vi "Climb_Motors.vi"(4 "Driver - Right Thumb":bool, 6 "Driver - Left Thumb":bool, 8 "Driver - Trigger":bool, 9 "Driver - Left Top left":bool, 10 "Driver - Right Top Right":bool) -> ()   [LabVIEW 2020]
uses:
  <vilib>/Rock Robotics/WPI/ThirdParty/Phoenix-LabVIEW/Motor Controller/Controls/CTRE_Phoenix_MotorControl_ControlMode.ctl
  <vilib>/Rock Robotics/Network Tables/NT Read String.vi
panel:
  in  "Traversal 2":dbl
  in  "Traversal 1":dbl
  in  "High 2":dbl
  in  "High 1":dbl
  in  "Mid 2":dbl=400000.0
  in  "Mid 1":dbl=400000.0
  in  "Low 2":dbl=150000.0
  in  "Low 1":dbl=150000.0
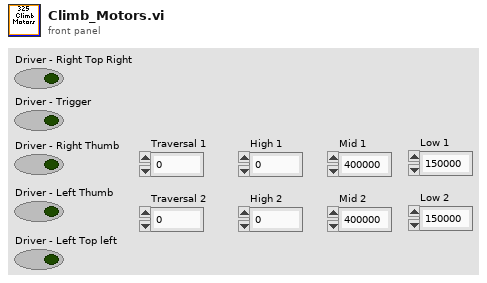
[diagram p1: front panel]
types:
  T1 = typedef "WPI_MotorControlDeviceRef.ctl" = cluster{"DeviceStatus":errorcluster, "Type":T2, "PWM":cluster{"PWM Channel":T3, "DeadBand":T4}, "CAN":cluster{"Device Number":u8, "SetOutput VI Ref":variant, "GetOutput VI Ref":variant, "Enable VI Ref":variant, "Disable VI Ref":variant, "Data":variant}, "Invert":bool, "DIO PWM":cluster{"PWM \"Enable\" Channel":T3, "DIOChannel":T5, "PWM Rate":dbl}}
  T2 = typedef "WPI_MotorControlType.ctl" = enum16{"PWM", "CAN", "DIO PWM"}
  T3 = typedef "FPGA_DIOPWMChannel.ctl" = enum8{"PWM 0", "PWM 1", "PWM 2", "PWM 3", "PWM 4", "PWM 5", "PWM 6", "PWM 7", "PWM 8", "PWM 9", "PWM MXP 0", "PWM MXP 1", "PWM MXP 2", "PWM MXP 3", "PWM MXP 4", "PWM MXP 5", "PWM MXP 6", "PWM MXP 7", "PWM MXP 8", "PWM MXP 9", "Invalid"}
  T4 = typedef "WPI_PWMDeadband.ctl" = cluster{"Name":string, "maxPositivePwm":i32, "minPositivePwm":i32, "centerPwm":i32, "maxNegativePwm":i32, "minNegativePwm":i32, "angularRange":u16}
  T5 = typedef "FPGA_DIOChannel.ctl" = enum8{"DIO 0", "DIO 1", "DIO 2", "DIO 3", "DIO 4", "DIO 5", "DIO 6", "DIO 7", "DIO 8", "DIO 9", "DIO MXP 0", "DIO MXP 1", "DIO MXP 2", "DIO MXP 3", "DIO MXP 4", "DIO MXP 5", "DIO MXP 6", "DIO MXP 7", "DIO MXP 8", "DIO MXP 9", "DIO MXP 10", "DIO MXP 11", "DIO MXP 12", "DIO MXP 13", "DIO MXP 14", "DIO MXP 15", "SPI Port CS1", "SPI Port CS2", "SPI Port CS3", "SPI Port MISO", "SPI Port MOSI", "Invalid"}
  T6 = typedef "CTRE_Phoenix_MotorControl_ControlMode.ctl" = u16
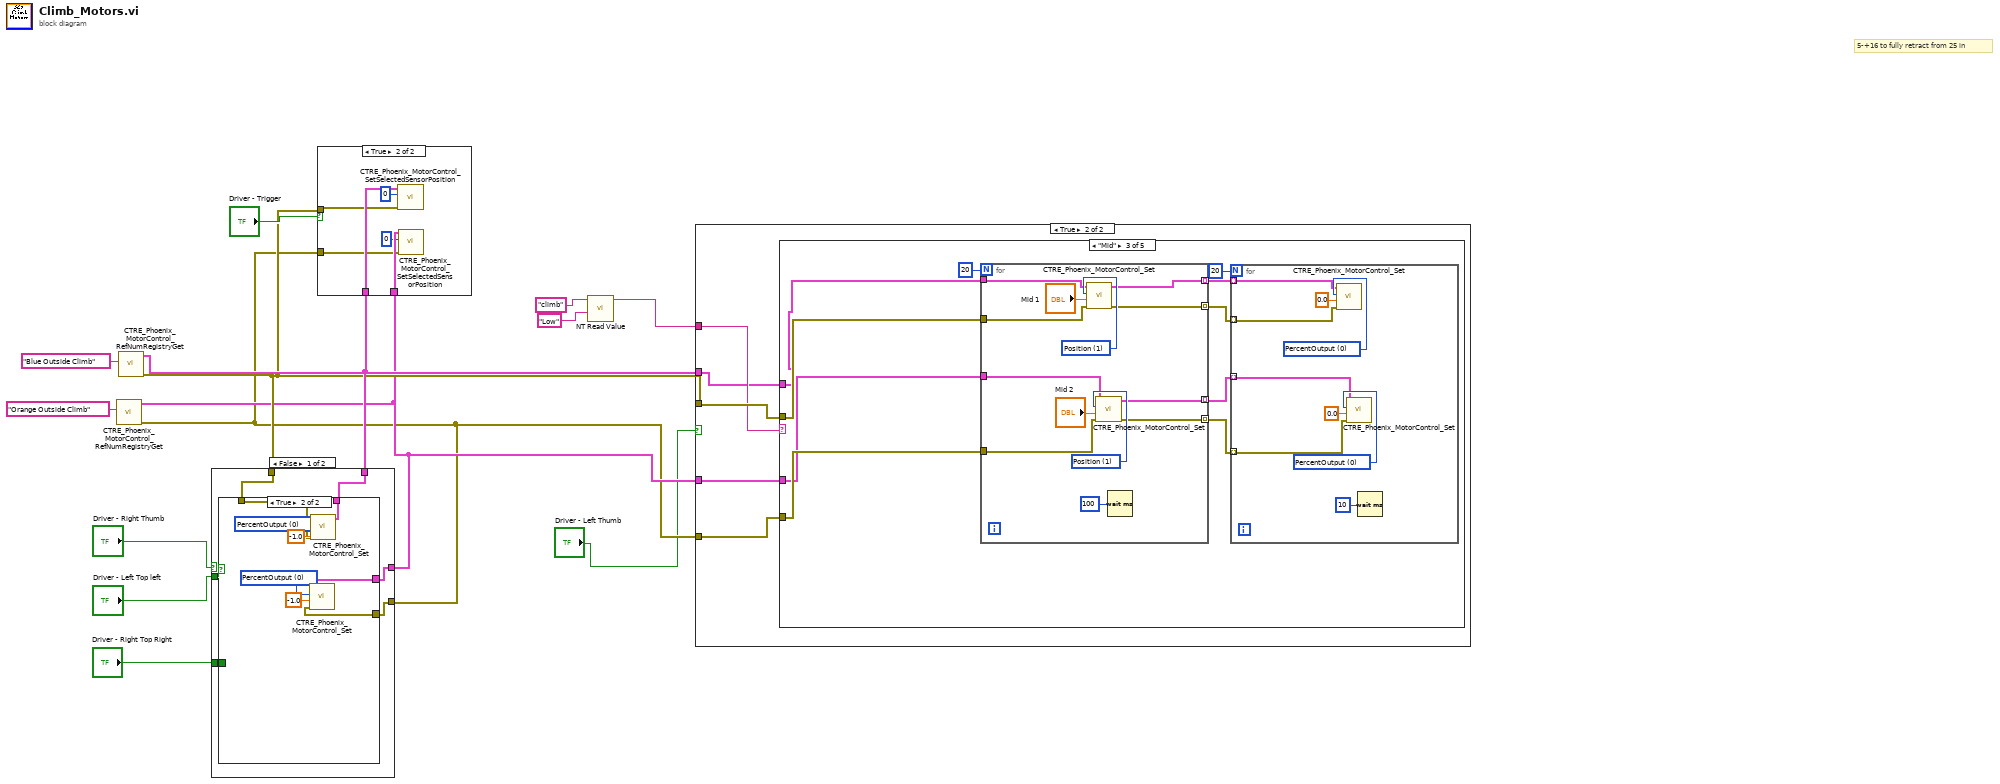
[diagram p0: block diagram]
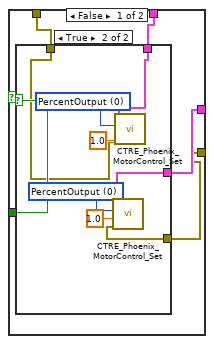
[diagram p2: hidden frame]
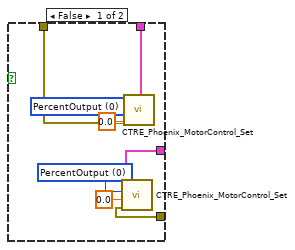
[diagram p3: hidden frame]
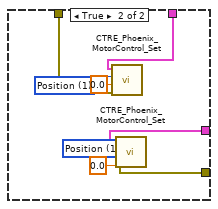
[diagram p4: hidden frame]
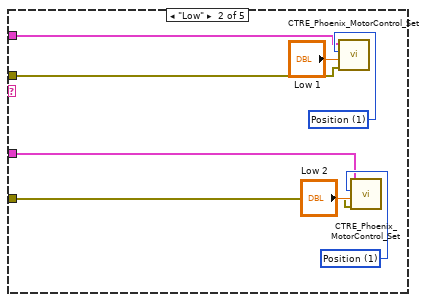
[diagram p7: hidden frame]
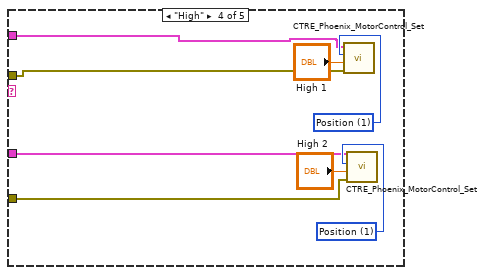
[diagram p8: hidden frame]
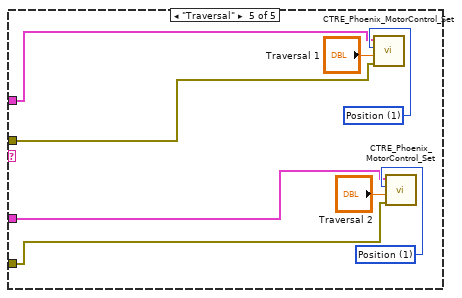
[diagram p9: hidden frame]
diagram:
  # "5-+16 to fully retract from 25 in"
  n1 = call <vilib>:"CTRE_Phoenix_MotorControl_RefNumRegistryGet.vi"("refnum name"="Orange Outside Climb") -> ("error out"=w7:errorcluster, "PhoenixMotorControlDevRef"=w8:T1)  [unwired: 9 in]
  n2 = call <vilib>:"CTRE_Phoenix_MotorControl_RefNumRegistryGet.vi"("refnum name"="Blue Outside Climb") -> ("error out"=w9:errorcluster, "PhoenixMotorControlDevRef"=w10:T1)  [unwired: 9 in]
  n3 = case shown="False" "Driver - Right Thumb" {
    tunnel: w10 -> [w19 w53]
    tunnel: w9 -> [w18 w52]
    tunnel: w8 -> [w17 w51]
    tunnel: w7 -> [w16 w50]
    tunnel: "Driver - Left Top left" -> [w20 _]
    tunnel: "Driver - Right Top Right" -> [w15 _]
    frame False {
      n4 = case shown="True" w20 {
        tunnel: w19 -> [w24 w45]
        tunnel: w18 -> [w23 w44]
        tunnel: w17 -> [w22 w43]
        tunnel: w16 -> [w21 w42]
        tunnel: w15 -> [w25 _]
        frame False {
          n5 = case shown="True" w25 {
            tunnel: w24 -> [w29 w34]
            tunnel: w23 -> [w28 w35]
            tunnel: w22 -> [w27 w36]
            tunnel: w21 -> [w26 w37]
            frame False {
              w32 = T6 0 items=["PercentOutput"=0, "Position"=1, "Velocity"=2, "Current"=3, "Follower"=5, "MotionProfile"=6, "MotionMagic"=7, "MotionProfileArc"=10, "Disabled"=15] ("Control Mode")
              w33 = T6 0 items=["PercentOutput"=0, "Position"=1, "Velocity"=2, "Current"=3, "Follower"=5, "MotionProfile"=6, "MotionMagic"=7, "MotionProfileArc"=10, "Disabled"=15] ("Control Mode")
              n6 = call <vilib>:"CTRE_Phoenix_MotorControl_Set.vi"("error in (no error)"=w26, "Output"=0.0, "Control Mode"=w33, "PhoenixMotorControlDevRef"=w27) -> ()  [unwired: 6 in, 2 out]
              n7 = call <vilib>:"CTRE_Phoenix_MotorControl_Set.vi"("error in (no error)"=w28, "Output"=0.0, "Control Mode"=w32, "PhoenixMotorControlDevRef"=w29) -> ()  [unwired: 6 in, 2 out]
            }
            frame True {
              w40 = T6 0 items=["PercentOutput"=0, "Position"=1, "Velocity"=2, "Current"=3, "Follower"=5, "MotionProfile"=6, "MotionMagic"=7, "MotionProfileArc"=10, "Disabled"=15] ("Control Mode")
              w41 = T6 0 items=["PercentOutput"=0, "Position"=1, "Velocity"=2, "Current"=3, "Follower"=5, "MotionProfile"=6, "MotionMagic"=7, "MotionProfileArc"=10, "Disabled"=15] ("Control Mode")
              n8 = call <vilib>:"CTRE_Phoenix_MotorControl_Set.vi"("error in (no error)"=w37, "Output"=1.0, "Control Mode"=w41, "PhoenixMotorControlDevRef"=w36) -> ()  [unwired: 6 in, 2 out]
              n9 = call <vilib>:"CTRE_Phoenix_MotorControl_Set.vi"("error in (no error)"=w35, "Output"=1.0, "Control Mode"=w40, "PhoenixMotorControlDevRef"=w34) -> ()  [unwired: 6 in, 2 out]
            }
          }
        }
        frame True {
          w48 = T6 0 items=["PercentOutput"=0, "Position"=1, "Velocity"=2, "Current"=3, "Follower"=5, "MotionProfile"=6, "MotionMagic"=7, "MotionProfileArc"=10, "Disabled"=15] ("Control Mode")
          w49 = T6 0 items=["PercentOutput"=0, "Position"=1, "Velocity"=2, "Current"=3, "Follower"=5, "MotionProfile"=6, "MotionMagic"=7, "MotionProfileArc"=10, "Disabled"=15] ("Control Mode")
          n10 = call <vilib>:"CTRE_Phoenix_MotorControl_Set.vi"("error in (no error)"=w42, "Output"=-1.0, "Control Mode"=w49, "PhoenixMotorControlDevRef"=w43) -> ()  [unwired: 6 in, 2 out]
          n11 = call <vilib>:"CTRE_Phoenix_MotorControl_Set.vi"("error in (no error)"=w44, "Output"=-1.0, "Control Mode"=w48, "PhoenixMotorControlDevRef"=w45) -> ()  [unwired: 6 in, 2 out]
        }
      }
    }
    frame True {
      w56 = T6 1 items=["PercentOutput"=0, "Position"=1, "Velocity"=2, "Current"=3, "Follower"=5, "MotionProfile"=6, "MotionMagic"=7, "MotionProfileArc"=10, "Disabled"=15] ("Control Mode")
      w57 = T6 1 items=["PercentOutput"=0, "Position"=1, "Velocity"=2, "Current"=3, "Follower"=5, "MotionProfile"=6, "MotionMagic"=7, "MotionProfileArc"=10, "Disabled"=15] ("Control Mode")
      n12 = call <vilib>:"CTRE_Phoenix_MotorControl_Set.vi"("error in (no error)"=w52, "Output"=0.0, "Control Mode"=w56, "PhoenixMotorControlDevRef"=w53) -> ()  [unwired: 6 in, 2 out]
      n13 = call <vilib>:"CTRE_Phoenix_MotorControl_Set.vi"("error in (no error)"=w50, "Output"=0.0, "Control Mode"=w57, "PhoenixMotorControlDevRef"=w51) -> ()  [unwired: 6 in, 2 out]
    }
  }
  n14 = case shown="True" "Driver - Trigger" {
    tunnel: w10 -> [_ w63]
    tunnel: w9 -> [_ w62]
    tunnel: w8 -> [_ w61]
    tunnel: w7 -> [_ w60]
    frame False {
    }
    frame True {
      n15 = call <vilib>:"CTRE_Phoenix_MotorControl_SetSelectedSensorPosition.vi"("error in (no error)"=w62, "New Sensor Position"=0, "PhoenixMotorControlDevRef"=w63) -> ()  [unwired: 7 in, 2 out]
      n16 = call <vilib>:"CTRE_Phoenix_MotorControl_SetSelectedSensorPosition.vi"("error in (no error)"=w60, "New Sensor Position"=0, "PhoenixMotorControlDevRef"=w61) -> ()  [unwired: 7 in, 2 out]
    }
  }
  n17 = call-poly <vilib>:"NT Read Value.vi"("Default Value"="Low", "Name"="climb") -> ("String"=w3:string)  [unwired: 8 in, 1 out]
  n18 = case shown="True" "Driver - Left Thumb" {
    tunnel: w10 -> [_ w64]
    tunnel: w9 -> [_ w68]
    tunnel: w8 -> [_ w67]
    tunnel: w7 -> [_ w66]
    tunnel: w3 -> [_ w65]
    frame False {
    }
    frame True {
      n19 = case shown="\"Mid\"" w65 {
        tunnel: w68 -> [_ w74 w86 w112 w120]
        tunnel: w67 -> [_ w71 w84 w111 w119]
        tunnel: w66 -> [_ w70 w85 w110 w118]
        tunnel: w64 -> [_ w69 w83 w109 w117]
        frame Default {
        }
        frame "Low" {
          w72 = T6 1 items=["PercentOutput"=0, "Position"=1, "Velocity"=2, "Current"=3, "Follower"=5, "MotionProfile"=6, "MotionMagic"=7, "MotionProfileArc"=10, "Disabled"=15] ("Control Mode")
          w75 = T6 1 items=["PercentOutput"=0, "Position"=1, "Velocity"=2, "Current"=3, "Follower"=5, "MotionProfile"=6, "MotionMagic"=7, "MotionProfileArc"=10, "Disabled"=15] ("Control Mode")
          n20 = call <vilib>:"CTRE_Phoenix_MotorControl_Set.vi"("error in (no error)"=w74, "Output"="Low 1", "Control Mode"=w75, "PhoenixMotorControlDevRef"=w69) -> ()  [unwired: 6 in, 2 out]
          n21 = call <vilib>:"CTRE_Phoenix_MotorControl_Set.vi"("error in (no error)"=w70, "Output"="Low 2", "Control Mode"=w72, "PhoenixMotorControlDevRef"=w71) -> ()  [unwired: 6 in, 2 out]
        }
        frame "Mid" {
          n22 = for {
            N: 20 -> [_]
            tunnel: w86 -> [w104]
            tunnel: w85 -> [w103]
            tunnel: w84 -> [w102]
            tunnel: w83 -> [w101]
            tunnel: [w99] -> w81 mode=indexing
            tunnel: [w98] -> w80 mode=indexing
            tunnel: [w97] -> w79 mode=indexing
            tunnel: [w96] -> w78 mode=indexing
            w105 = T6 1 items=["PercentOutput"=0, "Position"=1, "Velocity"=2, "Current"=3, "Follower"=5, "MotionProfile"=6, "MotionMagic"=7, "MotionProfileArc"=10, "Disabled"=15] ("Control Mode")
            w107 = T6 1 items=["PercentOutput"=0, "Position"=1, "Velocity"=2, "Current"=3, "Follower"=5, "MotionProfile"=6, "MotionMagic"=7, "MotionProfileArc"=10, "Disabled"=15] ("Control Mode")
            n23 = call <vilib>:"CTRE_Phoenix_MotorControl_Set.vi"("error in (no error)"=w104, "Output"="Mid 1", "Control Mode"=w107, "PhoenixMotorControlDevRef"=w101) -> ("error out"=w97:errorcluster, "PhoenixMotorControlDevRef"=w96:T1)  [unwired: 6 in]
            n24 = call <vilib>:"CTRE_Phoenix_MotorControl_Set.vi"("error in (no error)"=w103, "Output"="Mid 2", "Control Mode"=w105, "PhoenixMotorControlDevRef"=w102) -> ("error out"=w99:errorcluster, "PhoenixMotorControlDevRef"=w98:T1)  [unwired: 6 in]
            n25 = Wait (ms)(milliseconds to wait=u32 100) -> ()  [unwired: 1 out]
          }
          n26 = for {
            N: 20 -> [_]
            tunnel: w79 -> [w93] mode=indexing
            tunnel: w81 -> [w92] mode=indexing
            tunnel: w80 -> [w91] mode=indexing
            tunnel: w78 -> [w90] mode=indexing
            w94 = T6 0 items=["PercentOutput"=0, "Position"=1, "Velocity"=2, "Current"=3, "Follower"=5, "MotionProfile"=6, "MotionMagic"=7, "MotionProfileArc"=10, "Disabled"=15] ("Control Mode")
            w95 = T6 0 items=["PercentOutput"=0, "Position"=1, "Velocity"=2, "Current"=3, "Follower"=5, "MotionProfile"=6, "MotionMagic"=7, "MotionProfileArc"=10, "Disabled"=15] ("Control Mode")
            n27 = call <vilib>:"CTRE_Phoenix_MotorControl_Set.vi"("error in (no error)"=w93, "Output"=0.0, "Control Mode"=w95, "PhoenixMotorControlDevRef"=w90) -> ()  [unwired: 6 in, 2 out]
            n28 = call <vilib>:"CTRE_Phoenix_MotorControl_Set.vi"("error in (no error)"=w92, "Output"=0.0, "Control Mode"=w94, "PhoenixMotorControlDevRef"=w91) -> ()  [unwired: 6 in, 2 out]
            n29 = Wait (ms)(milliseconds to wait=u32 10) -> ()  [unwired: 1 out]
          }
        }
        frame "High" {
          w113 = T6 1 items=["PercentOutput"=0, "Position"=1, "Velocity"=2, "Current"=3, "Follower"=5, "MotionProfile"=6, "MotionMagic"=7, "MotionProfileArc"=10, "Disabled"=15] ("Control Mode")
          w115 = T6 1 items=["PercentOutput"=0, "Position"=1, "Velocity"=2, "Current"=3, "Follower"=5, "MotionProfile"=6, "MotionMagic"=7, "MotionProfileArc"=10, "Disabled"=15] ("Control Mode")
          n30 = call <vilib>:"CTRE_Phoenix_MotorControl_Set.vi"("error in (no error)"=w112, "Output"="High 1", "Control Mode"=w115, "PhoenixMotorControlDevRef"=w109) -> ()  [unwired: 6 in, 2 out]
          n31 = call <vilib>:"CTRE_Phoenix_MotorControl_Set.vi"("error in (no error)"=w110, "Output"="High 2", "Control Mode"=w113, "PhoenixMotorControlDevRef"=w111) -> ()  [unwired: 6 in, 2 out]
        }
        frame "Traversal" {
          w121 = T6 1 items=["PercentOutput"=0, "Position"=1, "Velocity"=2, "Current"=3, "Follower"=5, "MotionProfile"=6, "MotionMagic"=7, "MotionProfileArc"=10, "Disabled"=15] ("Control Mode")
          w123 = T6 1 items=["PercentOutput"=0, "Position"=1, "Velocity"=2, "Current"=3, "Follower"=5, "MotionProfile"=6, "MotionMagic"=7, "MotionProfileArc"=10, "Disabled"=15] ("Control Mode")
          n32 = call <vilib>:"CTRE_Phoenix_MotorControl_Set.vi"("error in (no error)"=w120, "Output"="Traversal 1", "Control Mode"=w123, "PhoenixMotorControlDevRef"=w117) -> ()  [unwired: 6 in, 2 out]
          n33 = call <vilib>:"CTRE_Phoenix_MotorControl_Set.vi"("error in (no error)"=w118, "Output"="Traversal 2", "Control Mode"=w121, "PhoenixMotorControlDevRef"=w119) -> ()  [unwired: 6 in, 2 out]
        }
      }
    }
  }
